vi "ILABs_CreateFromTemplate.vi"(2 "suffix":string, 3 "templateName":string, 4 "path":string, 5 "appRef":refnum<vi>) -> (0 "viReference":refnum<vi>, 1 "name":string)   [LabVIEW 2009]
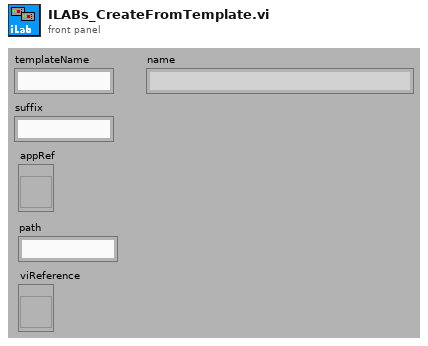
[diagram p1: front panel]
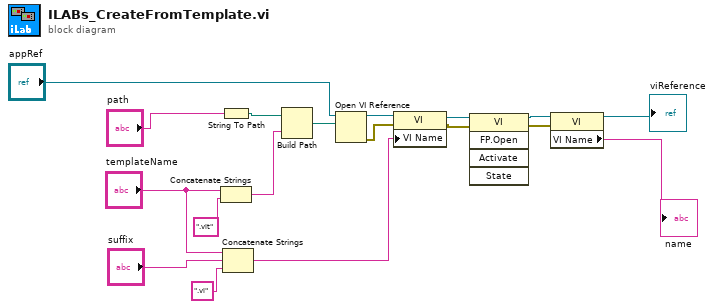
[diagram p0: block diagram]
diagram:
  n1 = String To Path(string="path") -> (path=w8:path)
  n2 = Concatenate Strings("templateName", ".vit" ("string")) -> (w12:string)
  n3 = Concatenate Strings("templateName", "suffix", ".vi" ("string")) -> (w11:string)
  n4 = Build Path(base path=w8, name or relative path=w12) -> (appended path=w10:path)
  n5 = Open VI Reference(application reference (local)="appRef", vi path=w10) -> (vi reference=w18:refnum<vi>, error out=w17:errorcluster)  [unwired: 1 in, 3 out]
  n6 = property class="VI"(reference=w18, error in=w17, "VI Name"=w11) -> (reference out=w3:refnum<vi>, error out=w1:errorcluster)
  n7 = invoke class="VI" method="FP.Open"(reference=w3, error in=w1) -> (reference out=w4:refnum<vi>, error out=w2:errorcluster)  [unwired: 3 in, 3 out]
  n8 = property class="VI"(reference=w4, error in=w2) -> (reference out=→"viReference":refnum<vi>, "VI Name"=→"name":string)  [unwired: 1 out]
